vi "Pupulate and conf serial bus.vi"(8 "Error In":errorcluster, 9 "Empty buffer":bool) -> (0 "Error Out":errorcluster, 3 "Devices":refnum<visa-resource-name>[](array[refnum]))   [LabVIEW 2021]
uses:
  <vilib>/Instr/_visa.llb/VISA Find Search Mode.ctl
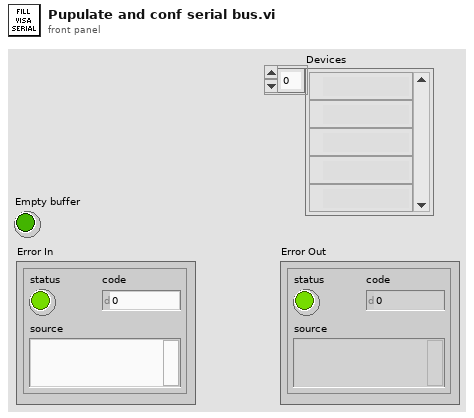
[diagram p1: front panel]
types:
  T1 = typedef "VISA Find Search Mode.ctl" = u32
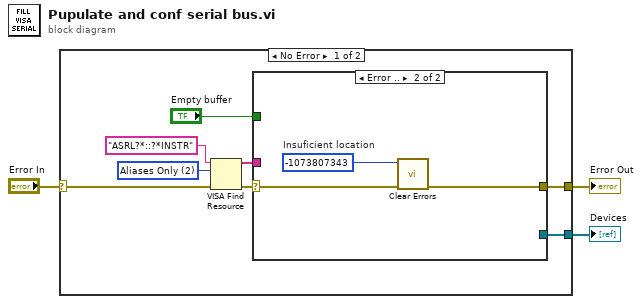
[diagram p0: block diagram]
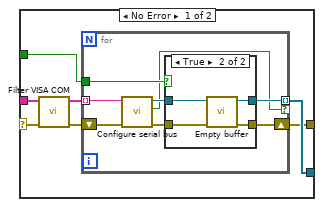
[diagram p2: hidden frame]
diagram:
  n1 = case shown="No Error" "Error In" {
    selector: "Error In" -> [w5 w36]
    tunnel: [w9 _] -> w3
    tunnel: [w8 w36] -> w2
    frame No Error {
      w11 = T1 2 items=["Canonical Names Only"=0, "Aliases Only"=2, "Include Matching Aliases"=3, "Include All Aliases"=4] ("Search Mode")
      n2 = VISA Find Resource(8:w5, 10:w11, 11:"ASRL?*::?*INSTR" ("expression (\"?*\")")) -> (0:w4:errorcluster, 3:w6:string[])  [unwired: 1 out]
      n3 = case shown="Error .." w4 {
        selector: w4 -> [w12 w35]
        tunnel: [w18 _] -> w9
        tunnel: [w17 w34] -> w8
        tunnel: "Empty buffer" -> [w16 _]
        tunnel: w6 -> [w15 _]
        frame No Error {
          n4 = call "Filter VISA COM.vi"("Error In"=w12, "Names in"=w15) -> ("Error Out"=w13:errorcluster, "COM only list"=w14:string[])  [unwired: 7 in, 1 out]
          n5 = for {
            tunnel: w14 -> [w26] mode=indexing
            tunnel: [w20] -> w18 mode=indexing if=w19
            shift-right: [w22] -> w17
            shift-left: w13 -> [w25]
            tunnel: w16 -> [w24]
            n6 = call "Configure serial bus.vi"("Error In"=w25, "VISA resource name"=w26) -> ("Error Out"=w23:errorcluster, "Add instrument"=w19:bool, "VISA resource name 2"=w21:refnum<visa-resource-name>)  [unwired: 7 in]
            n7 = case shown="True" w24 {
              tunnel: w23 -> [w27 w32]
              tunnel: [w27 w31] -> w22
              tunnel: w21 -> [w28 w30]
              tunnel: [w28 w29] -> w20
              frame False {
              }
              frame True {
                n8 = call "Empty buffer.vi"("Error In"=w32, "VISA resource name"=w30) -> ("Error Out"=w31:errorcluster, "VISA resource name out"=w29:refnum<visa-resource-name>)  [unwired: 7 in, 1 out]
              }
            }
          }
        }
        frame Error {
          w33 = -1073807343  # Insuficient location
          n9 = call <vilib>:"Clear Errors.vi"("error in (no error)"=w35, "specific error code to clear (0: all)"=w33) -> ("error out"=w34:errorcluster)  [unwired: 4 in, 1 out]
        }
      }
    }
    frame Error {
    }
  }
  "Devices" <- w3
  "Error Out" <- w2
